vi "SmartMotor_InitializeMotors.vi"(8 "error in (no error)":errorcluster, 9 "ReadWait":u32=50, 10 "MotorInitCmds":string[](array[string]), 11 "VISA In":refnum<visa-resource-name>) -> (0 "error out":errorcluster, 2 "cmd str out":string, 3 "VISA Out":refnum<visa-resource-name>)   [LabVIEW 2017]
uses:
  TD SerialBusMotorSpecifier_enum.ctl
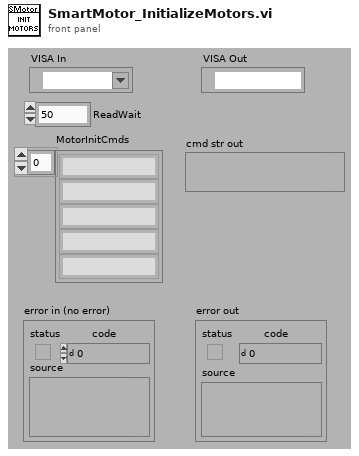
[diagram p1: front panel]
types:
  T1 = typedef "TD SerialBusMotorSpecifier_enum.ctl" = enum16{"None", "Global", "M1", "M2", "M3"}
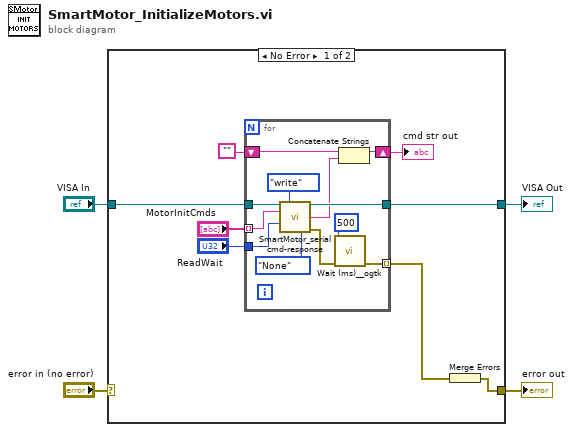
[diagram p0: block diagram]
diagram:
  n1 = case shown="No Error" "error in (no error)" {
    selector: "error in (no error)" -> [_ w26]
    tunnel: "VISA In" -> [w12 w25]
    tunnel: [w9 w26] -> w3
    tunnel: [w11 w25] -> w2
    frame No Error {
      n2 = for {
        tunnel: w12 -> [w23]
        tunnel: [w22] -> w11
        tunnel: [w19] -> w10 mode=indexing
        tunnel: "MotorInitCmds" -> [w21] mode=indexing
        shift-right: [w15] -> w6
        shift-left: "" -> [w16]
        tunnel: "ReadWait" -> [w13]
        n3 = call "SmartMotor_serial cmd-response.vi"("VISA In"=w23, "mode"=enum16{"wr & rd", "write", "read"}."write", "cmd"=w21, "ReadWait"=w13, "MotorSpecifier(None)"=TD_SerialBusMotorSpecifier_enum."None" ("MotorSpecifier(M1)")) -> ("VISA out"=w22:refnum<visa-resource-name>, "cmd str out"=w14:string, "error out"=w20:errorcluster)  [unwired: 6 in, 2 out]
        n4 = call <userlib>:"Wait (ms)__ogtk.vi"("error in (no error)"=w20, "milliseconds to wait"=u32 500 ("Read wait (ms)")) -> ("error out"=w19:errorcluster)  [unwired: 8 in, 1 out]
        n5 = Concatenate Strings(w16, w14) -> (w15:string)
      }
      "cmd str out" <- w6
      n6 = Merge Errors(w10) -> (w9:errorcluster)
    }
    frame Error {
    }
  }
  "VISA Out" <- w2
  "error out" <- w3
